vi "acender_led_push_button_potenciometro.vi"() -> ()   [LabVIEW 2018]
uses:
  <vilib>/Instr/_visa.llb/VISA Configure Serial Port (Instr).vi
panel:
  in  "OK Button":bool
  in  "Boolean 2":bool
  out "Meter":dbl(knob) scale=0.0..1023.0
  out "Boolean":bool
  in  "VISA resource name":refnum<visa-resource-name>
  in  "stop":bool
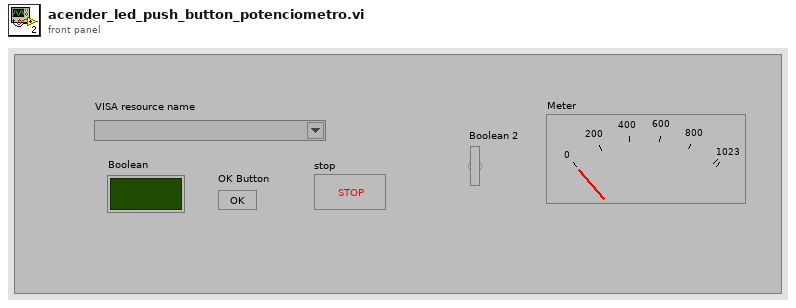
[diagram p1: front panel]
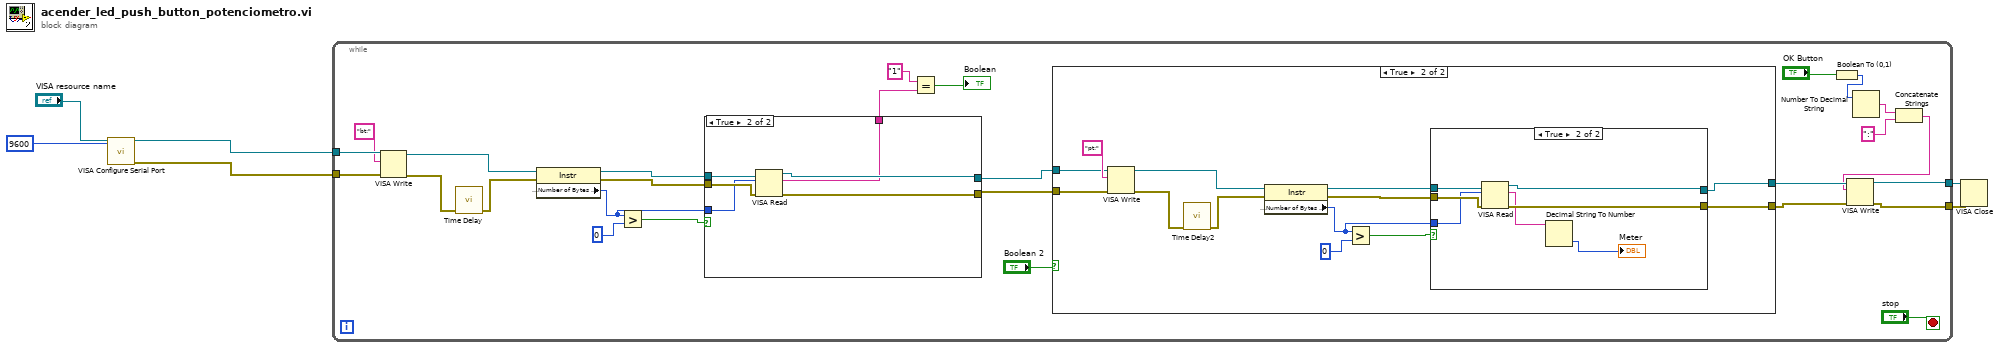
[diagram p0: block diagram]
diagram:
  n1 = call-poly "VISA Configure Serial Port"("VISA resource name"="VISA resource name", "baud rate (9600)"=u32 9600) -> ("VISA resource name out"=w4:refnum<visa-resource-name>, "error out"=w3:errorcluster)  [unwired: 12 in]
  n2 = while {
    tunnel: w4 -> [w32]
    tunnel: w3 -> [w31]
    tunnel: [w10] -> w1
    tunnel: [w11] -> w2
    stop <- "stop" stop-if-true
    n3 = VISA Write(VISA resource name=w32, write buffer="bt:", error in (no error)=w31) -> (VISA resource name out=w28:refnum<visa-resource-name>, error out=w30:errorcluster)  [unwired: 1 out]
    n4 = call "Time Delay"("error in (no error)"=w30) -> ("error out"=w27:errorcluster)  [unwired: 10 in]
    n5 = property class="Instr"(reference=w28, error in=w27) -> (reference out=w24:refnum<visa-resource-name>, error out=w23:errorcluster, "Serial Settings:Number of Bytes at Serial Port"=w22:u32)
    n6 = Greater?(x=w22, y=u32 0) -> (0:w26:bool)
    n7 = case shown="True" w26 {
      tunnel: w24 -> [w59 w65]
      tunnel: w23 -> [w58 w64]
      tunnel: w22 -> [_ w63]
      tunnel: [w59 w62] -> w18
      tunnel: [w58 w61] -> w17
      tunnel: [_ w60] -> w21
      frame False {
      }
      frame True {
        n8 = VISA Read(VISA resource name=w65, byte count=w63, error in (no error)=w64) -> (VISA resource name out=w62:refnum<visa-resource-name>, read buffer=w60:string, error out=w61:errorcluster)  [unwired: 1 out]
      }
    }
    n9 = Equal?(x="1", y=w21) -> (x = y?=→"Boolean":bool)
    n10 = case shown="True" "Boolean 2" {
      tunnel: w18 -> [w35 w39]
      tunnel: w17 -> [w34 w38]
      tunnel: [w35 w37] -> w13
      tunnel: [w34 w36] -> w12
      frame False {
      }
      frame True {
        n11 = VISA Write(VISA resource name=w39, write buffer="pt:", error in (no error)=w38) -> (VISA resource name out=w46:refnum<visa-resource-name>, error out=w48:errorcluster)  [unwired: 1 out]
        n12 = call "Time Delay2"("error in (no error)"=w48) -> ("error out"=w45:errorcluster)  [unwired: 10 in]
        n13 = property class="Instr"(reference=w46, error in=w45) -> (reference out=w42:refnum<visa-resource-name>, error out=w41:errorcluster, "Serial Settings:Number of Bytes at Serial Port"=w40:u32)
        n14 = Greater?(x=w40, y=u32 0) -> (0:w44:bool)
        n15 = case shown="True" w44 {
          tunnel: w42 -> [w50 w57]
          tunnel: w41 -> [w49 w56]
          tunnel: w40 -> [_ w55]
          tunnel: [w50 w54] -> w37
          tunnel: [w49 w53] -> w36
          frame False {
          }
          frame True {
            n16 = VISA Read(VISA resource name=w57, byte count=w55, error in (no error)=w56) -> (VISA resource name out=w54:refnum<visa-resource-name>, read buffer=w51:string, error out=w53:errorcluster)  [unwired: 1 out]
            n17 = Decimal String To Number(string=w51) -> (number=→"Meter":i32)  [unwired: 2 in, 1 out]
          }
        }
      }
    }
    n18 = Boolean To (0,1)(Boolean="OK Button") -> (0, 1=w15:i16)
    n19 = Number To Decimal String(number=w15) -> (decimal integer string=w9:string)  [unwired: 1 in]
    n20 = Concatenate Strings(w9, ":" ("string")) -> (w7:string)
    n21 = VISA Write(VISA resource name=w13, write buffer=w7, error in (no error)=w12) -> (VISA resource name out=w10:refnum<visa-resource-name>, error out=w11:errorcluster)  [unwired: 1 out]
  }
  n22 = VISA Close(VISA resource name=w1, error in (no error)=w2) -> ()  [unwired: 1 out]
